vi "getPixelData.vi"(8 "error in (no error)":errorcluster, 11 "ax5 in":refnum<class "ax5.lvclass">) -> (0 "error out":errorcluster, 1 "Temp":dbl[][](array[numeric]), 2 "Image Pixels (U16)":u16[][](array[numeric]), 3 "ax5 out":refnum<class "ax5.lvclass">, 5 "Image Type":u32(ring) items=["Grayscale (U8)", "Grayscale (I16)", "Grayscale (SGL)", "Complex (CSG)", "RGB (U32)", "HSL (U32)", "RGB (U64)", "Grayscale (U16)"])   [LabVIEW 2017, in "ax5.lvclass"]
uses:
  ax5.lvclass
  \\psf\Home/Desktop/Elkhorn Test/Elkhorn Test/JSONRPC Server Framework Examples/builds/JSON RPC over TCP/RT CompactRIO Target/My Source Distribution/home/lvuser/natinst/bin/methods/camera.lvclass
  <resource>/objmgr/IMAQImage.rc
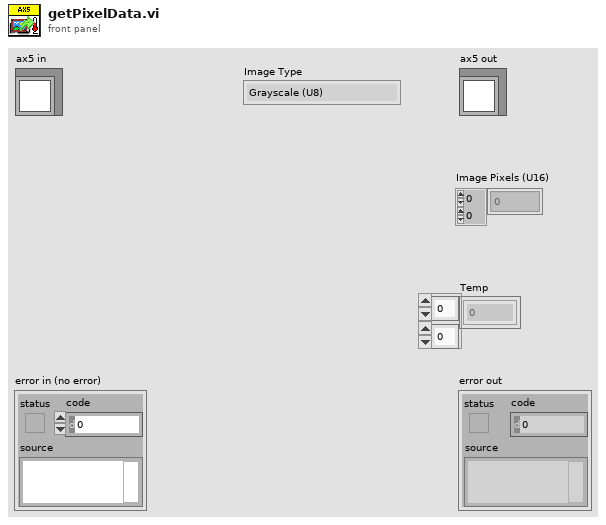
[diagram p1: front panel]
types:
  T1 = typedef "IMAQ Image.ctl" = refnum<image>
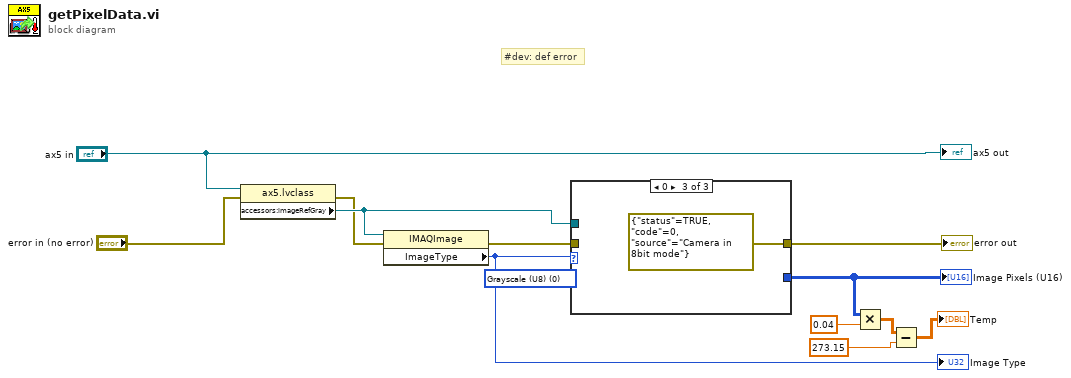
[diagram p0: block diagram]
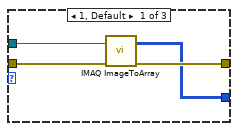
[diagram p2: hidden frame]
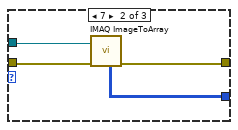
[diagram p3: hidden frame]
diagram:
  (unwired) u32 0 items=["Grayscale (U8)", "Grayscale (I16)", "Grayscale (SGL)", "Complex (CSG)", "RGB (U32)", "HSL (U32)", "RGB (U64)", "Grayscale (U16)"] ("Image Type")
  # "#dev: def error"
  n1 = property class="ax5.lvclass"(reference="ax5 in", error in="error in (no error)") -> (error out=w11:errorcluster, "accessors:imageRefGray"=w12:T1)  [unwired: 1 out]
  n2 = property class="IMAQImage"(reference=w12, error in=w11) -> (error out=w10:errorcluster, "ImageType"=w8:u32)  [unwired: 1 out]
  "Image Type" <- w8
  n3 = case shown="0" w8 {
    tunnel: w10 -> [w16 w20 _]
    tunnel: w12 -> [w15 w18 _]
    tunnel: [w13 w17 _] -> w6
    tunnel: [w14 w19 errorcluster {"status"=TRUE, "code"=0, "source"="Camera in 8bit mode"} ("error out")] -> w7
    frame 1, Default {
      n4 = call "IMAQ ImageToArray"("error in (no error)"=w16, "Image"=w15) -> ("error out"=w14:errorcluster, "Image Pixels (I16)"=w13:i16[][])  [unwired: 2 in, 3 out]
    }
    frame 7 {
      n5 = call "IMAQ ImageToArray"("error in (no error)"=w20, "Image"=w18) -> ("Image Pixels (U16)"=w17:u16[][], "error out"=w19:errorcluster)  [unwired: 2 in, 3 out]
    }
    frame 0 {
    }
  }
  "error out" <- w7
  "Image Pixels (U16)" <- w6
  n6 = Multiply(x=w6, y=0.04) -> (x*y=w4:dbl[][])
  n7 = Subtract(x=w4, y=273.15) -> (x-y=→"Temp":dbl[][])
  "ax5 out" <- "ax5 in"
